vi "sortFlies.vi"() -> ()   [LabVIEW 2012]
uses:
  image acquisition/GlobalBaslerCamera.vi
panel:
  out "selected path":path
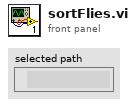
[diagram p1: front panel]
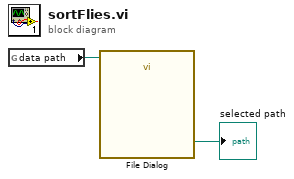
[diagram p0: block diagram]
diagram:
  n1 = global read "GlobalBaslerCamera.vi" "data path"() -> (w1:path)
  n2 = call "File Dialog"("start path"=w1) -> ("selected path"=→"selected path":path)  [unwired: 11 in, 3 out]
